vi "sec_Error_main.vi"(7 "Command (Check Error)":T3=enum."Check Error", 8 "error in (no error)":errorcluster, 10 "Error Event Refnum":T1, 11 "Process Loop Queue Refnum":T2) -> (0 "error out":errorcluster)   [LabVIEW 2009]
doc: "This Module is responsible for stopping the application when an error occurs.\nIt will signal the Event Loop via a User Event to shutdown and will flush and Shutdown the Main Loop."
uses:
  sec_Error_Command_enum.ctl
  controls/sec_ConsumerQueue_refnum.ctl
  controls/sec_ConsumerDataType_cluster.ctl
  controls/sec_ConsumerCommand_enum.ctl
  controls/sec_ErrorUserEventQueue_refnum.ctl
panel:
  # "Inputs"
  # "Outputs"
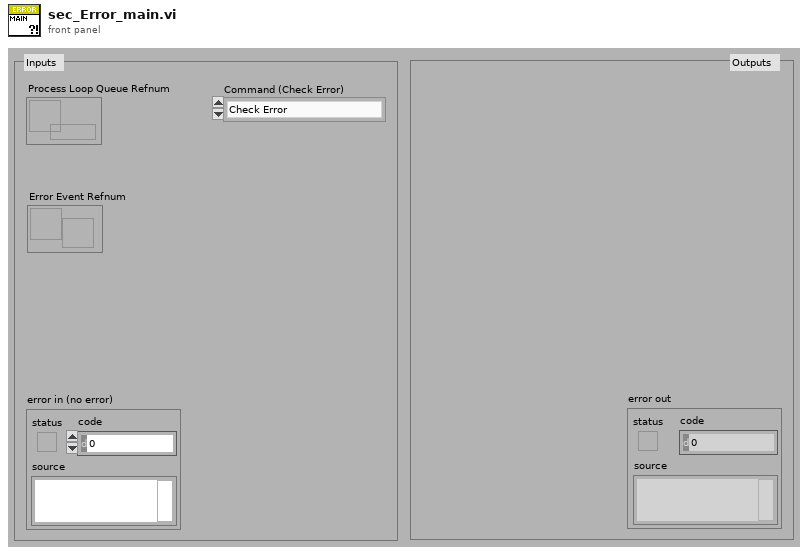
[diagram p1: front panel]
types:
  T1 = typedef "sec_ErrorUserEventQueue_refnum.ctl" = refnum<user-event>
  T2 = typedef "sec_ConsumerQueue_refnum.ctl" = refnum<queue>
  T3 = typedef "sec_Error_Command_enum.ctl" = enum16{"Initialise", "Check Error", "Report Errors"}
  T4 = typedef "sec_ConsumerDataType_cluster.ctl" = cluster{"Command":T5, "Data":variant}
  T5 = typedef "sec_ConsumerCommand_enum.ctl" = enum16{"Initialise", "Get Front Panel Data", "Set Front Panel Data", "Switch Updated", "Shutdown"}
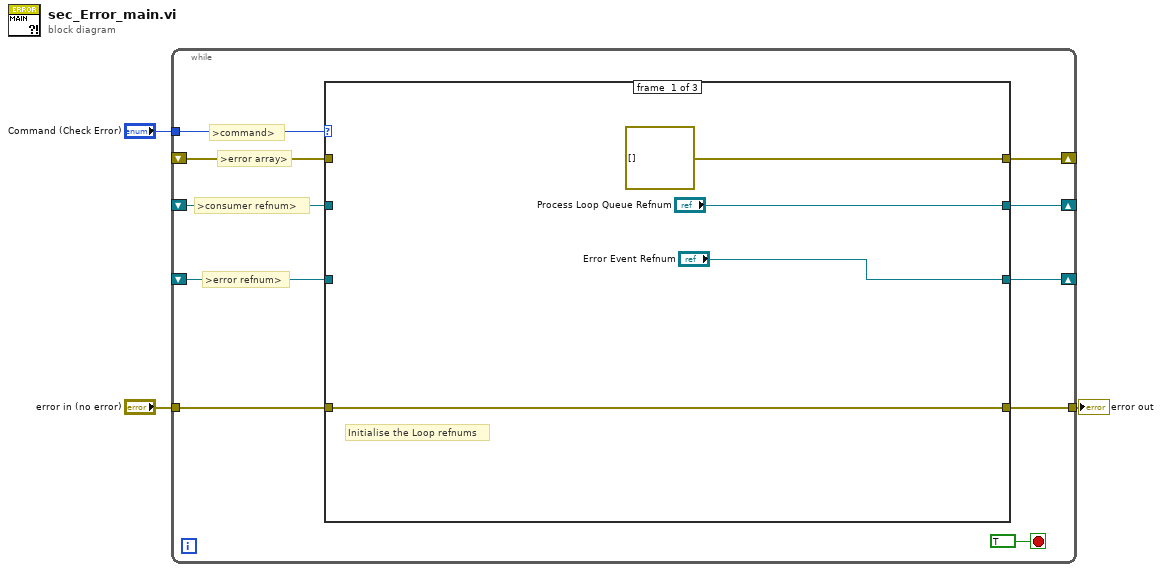
[diagram p0: block diagram]
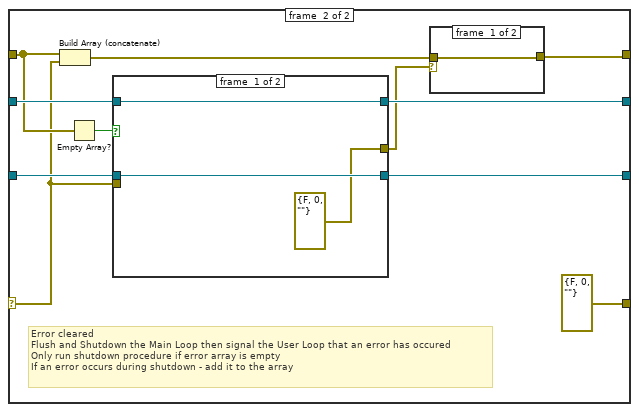
[diagram p3: hidden frame]
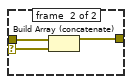
[diagram p4: hidden frame]
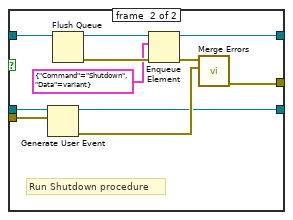
[diagram p5: hidden frame]
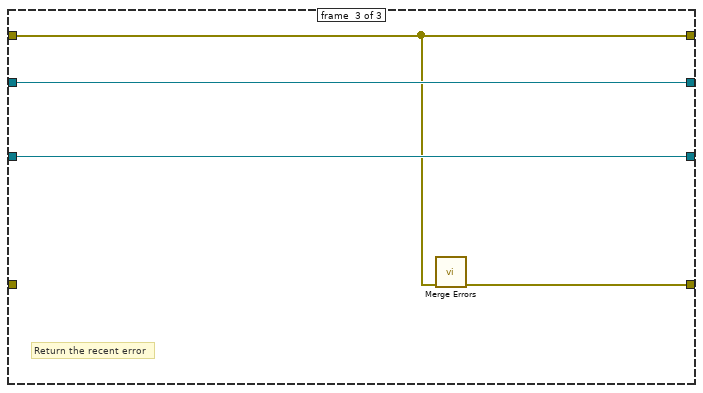
[diagram p6: hidden frame]
diagram:
  n1 = while {
    tunnel: [w13] -> w2
    tunnel: "error in (no error)" -> [w12]
    tunnel: "Command (Check Error)" -> [w11]
    shift-right: [w10] -> _
    shift-left: _ -> [w9]
    shift-right: [w7] -> _
    shift-left: _ -> [w6]
    shift-right: [w5] -> _
    shift-left: _ -> [w4]
    stop <- TRUE stop-if-true
    # ">error array>"
    # ">consumer refnum>"
    # ">error refnum>"
    # ">command>"
    n2 = case shown="\"Check Error\"" w11 {
      tunnel: [w17 w24 w59] -> w13
      tunnel: w12 -> [w17 w25 _]
      tunnel: ["Process Loop Queue Refnum" w21 w62] -> w10
      tunnel: w9 -> [_ w23 w62]
      tunnel: ["Error Event Refnum" w20 w61] -> w7
      tunnel: w6 -> [_ w22 w61]
      tunnel: [errorcluster[] [] w19 w60] -> w5
      tunnel: w4 -> [_ w18 w60]
      frame #0 {
        # "Initialise the Loop refnums"
      }
      frame #1 {
        n3 = case shown="Error" w25 {
          selector: w25 -> [w29 w30]
          tunnel: [w29 errorcluster {"status"=FALSE, "code"=0, "source"=""} ("error IO")] -> w24
          tunnel: w23 -> [w28 w39]
          tunnel: w22 -> [w27 w40]
          tunnel: [w28 w35] -> w21
          tunnel: [w27 w34] -> w20
          tunnel: [w26 w31] -> w19
          tunnel: w18 -> [w26 w38]
          frame #0 {
            # "No Error - Do nothing"
          }
          frame #1 {
            # "Error cleared\nFlush and Shutdown the Main Loop then signal the User Loop that an error has occured\nOnly run shutdown procedure if error array is empty\nIf an error occurs during shutdown - add it to the array"
            n4 = Build Array (concatenate)(w38, w30) -> (w33:errorcluster[])
            n5 = Empty Array?(array=w38) -> (empty?=w37:bool)
            n6 = case shown="True" w37 {
              tunnel: w40 -> [w46 w53]
              tunnel: w39 -> [w47 w54]
              tunnel: [errorcluster {"status"=FALSE, "code"=0, "source"=""} ("error out") w51] -> w32
              tunnel: [w47 w50] -> w35
              tunnel: [w46 w49] -> w34
              tunnel: w30 -> [_ w48]
              frame #0 {
              }
              frame #1 {
                # "Run Shutdown procedure"
                n7 = Generate User Event(user event=w53, event data cluster=w48) -> (user event out=w49:T1, error out=w52:errorcluster)  [unwired: 1 in]
                n8 = Flush Queue(queue=w54) -> (queue out=w57:T2, error out=w58:errorcluster)  [unwired: 1 in, 1 out]
                n9 = Enqueue Element(queue=w57, element=T4 {"Command"=enum."Shutdown", "Data"=variant}, error in (no error)=w58) -> (queue out=w50:T2, error out=w55:errorcluster)  [unwired: 1 in, 1 out]
                n10 = call <vilib>:"Merge Errors.vi"("error in 2 (no error)"=w52, "error in 1 (no error)"=w55) -> ("error out"=w51:errorcluster)  [unwired: 5 in]
              }
            }
            n11 = case shown="Error" w32 {
              selector: w32 -> [_ w42]
              tunnel: w33 -> [w41 w44]
              tunnel: [w41 w43] -> w31
              frame #0 {
              }
              frame #1 {
                n12 = Build Array (concatenate)(w44, w42) -> (w43:errorcluster[])
              }
            }
          }
        }
      }
      frame #2 {
        # "Return the recent error"
        n13 = call <vilib>:"Merge Errors.vi"("error array in"=w60) -> ("error out"=w59:errorcluster)  [unwired: 6 in]
      }
    }
  }
  "error out" <- w2
